vi "Solve1.vi"(8 "Error In":errorcluster, 11 "object in":refnum<class "2024_18.lvclass">) -> (0 "Error Out":errorcluster, 2 "Result":u64, 3 "object out":refnum<class "2024_18.lvclass">)   [LabVIEW 2023, in "2024_18.lvclass"]
uses:
  2024_18.lvclass
  2024_18.lvclass/2024_18.ctl
  Tile18.ctl
panel:
  out "NotFound":bool
  out "map":T1[][](array[typedef])
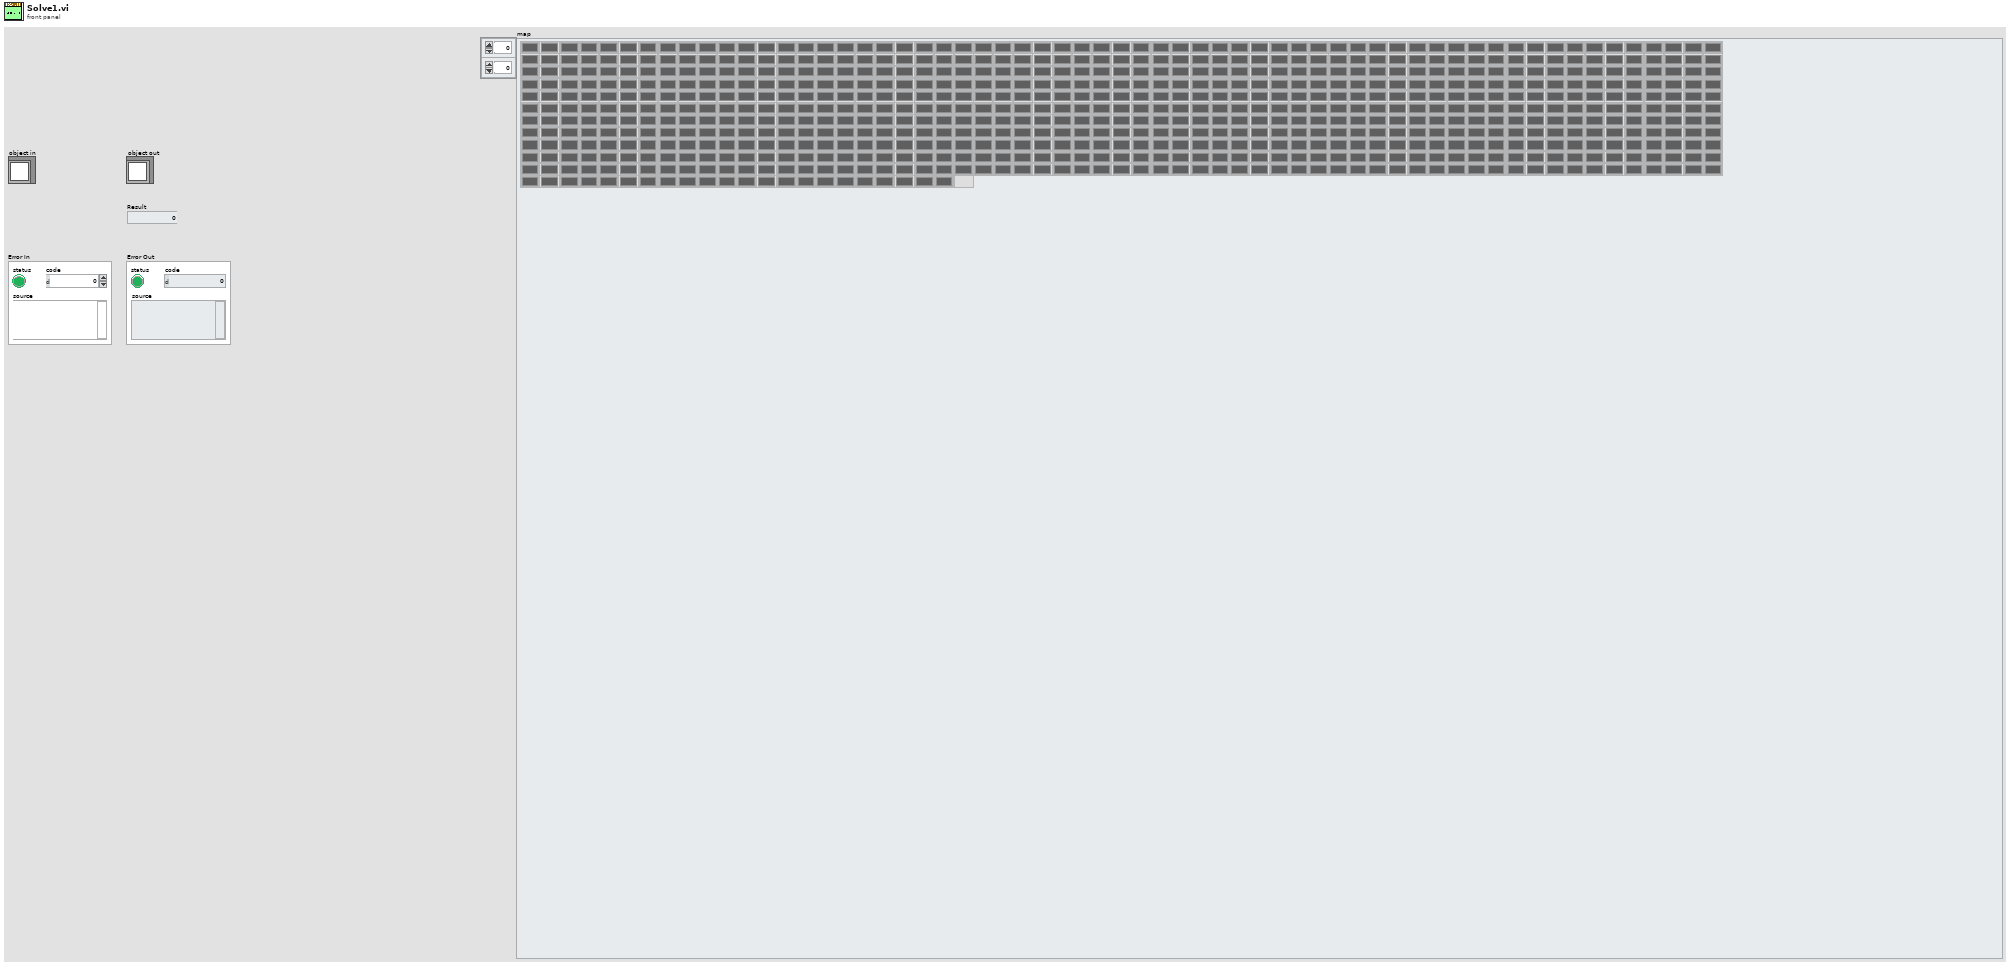
[diagram p1: front panel]
types:
  T1 = typedef "2024_18.lvclass/Tile18.ctl" = cluster{"Cost":i32, "BGColor":u32}
  T2 = typedef "AOC_XY(I32).ctl" = cluster{"X":i32, "Y":i32}
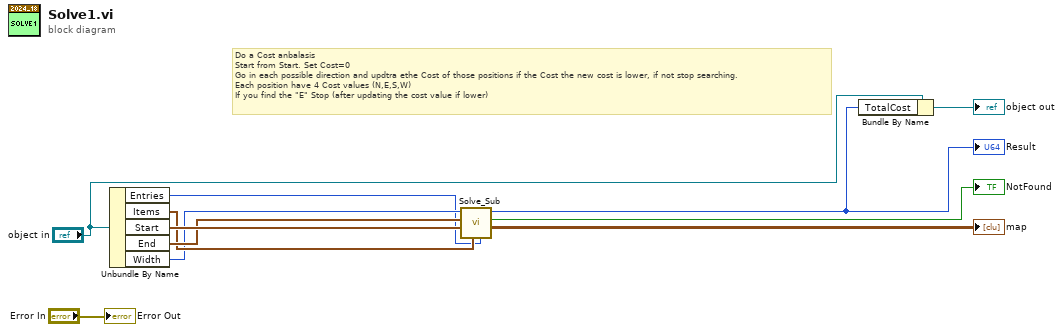
[diagram p0: block diagram]
diagram:
  # "Do a Cost anbalasis\nStart from Start. Set Cost=0\nGo in each possible direction and updtra ethe Cost of those positions if the Cost the new cost is lower, if not stop searching.\nEach position have 4 Cost values (N,E,S,W)\nIf you find the \"E\" Stop (after updating the cost value if lower)"
  n1 = Unbundle By Name("object in") -> ("Entries"=w3:i32, "Items"=w5:T2[], "Start"=w9:T2, "End"=w8:T2, "Width"=w4:i32)
  n2 = call "Solve_Sub.vi"("Entries"=w3, "Items"=w5, "Start"=w9, "End"=w8, "Width/Height"=w4) -> ("map"=→"map":T1[][], "key not found?"=→"NotFound":bool, "Cost"=w6:u64)  [unwired: 4 in]
  "Result" <- w6
  n3 = Bundle By Name(cluster="object in", "TotalCost"=w6) -> (→"object out":refnum<class "2024_18.lvclass">)
  "Error Out" <- "Error In"
